vi "GetROSfromTopic.vi"(0 "Topic":string) -> (2 "ROS":T1, 3 "Nice Name":string, 4 "Node?":bool)   [LabVIEW 2016]
doc: "Gets ROS typdef from the topic name"
uses:
  _ROSControl.ctl
  _ROSDirection.ctl
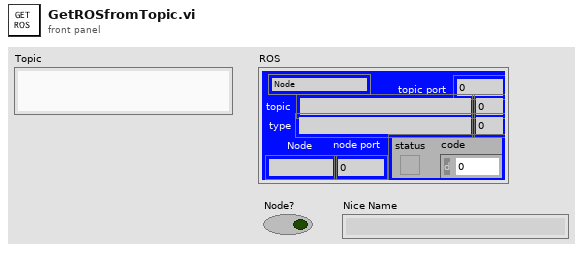
[diagram p1: front panel]
types:
  T1 = typedef "_ROSControl.ctl" = cluster{"topic port":u16, "Node":string, "topic":string, "type":string, "node port":u16, "error ":errorcluster, "Direction":T2, "Update (ms)":u16, "FIFO size":u16}
  T2 = typedef "_ROSDirection.ctl" = enum16{"Node", "Publisher", "Subscriber", "ServiceClient", "ServiceProvider"}
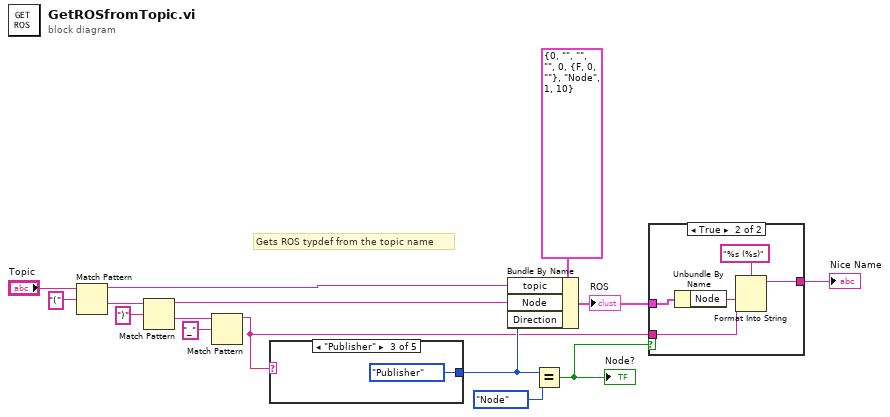
[diagram p0: block diagram]
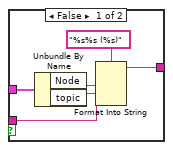
[diagram p2: hidden frame]
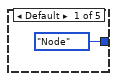
[diagram p3: hidden frame]
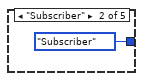
[diagram p4: hidden frame]
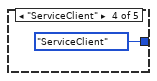
[diagram p5: hidden frame]
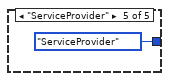
[diagram p6: hidden frame]
diagram:
  # "Gets ROS typdef from the topic name"
  n1 = Match Pattern(string="Topic", regular expression="(") -> (before substring=w5:string, after substring=w12:string)  [unwired: 1 in, 2 out]
  n2 = Match Pattern(string=w12, regular expression=")") -> (before substring=w6:string, after substring=w10:string)  [unwired: 1 in, 2 out]
  n3 = Match Pattern(string=w10, regular expression="_") -> (before substring=w4:string)  [unwired: 1 in, 3 out]
  n4 = case shown="\"Publisher\"" w4 {
    tunnel: [_ROSDirection."Node" ("Direction") _ROSDirection."Subscriber" ("Direction") _ROSDirection."Publisher" ("Direction") _ROSDirection."ServiceClient" ("Direction") _ROSDirection."ServiceProvider" ("Direction")] -> w8
    frame Default {
    }
    frame "Subscriber" {
    }
    frame "Publisher" {
    }
    frame "ServiceClient" {
    }
    frame "ServiceProvider" {
    }
  }
  n5 = Bundle By Name(cluster=T1 {"topic port"=0, "Node"="", "topic"="", "type"="", "node port"=0, "error "={"status"=FALSE, "code"=0, "source"=""}, "Direction"=enum."Node", "Update (ms)"=1, "FIFO size"=10} ("ROS"), "topic"=w5, "Node"=w6, "Direction"=w8) -> (w2:T1)
  "ROS" <- w2
  n6 = Equal?(x=w8, y=_ROSDirection."Node" ("Direction")) -> (x = y?=w1:bool)
  "Node?" <- w1
  n7 = case shown="True" w1 {
    tunnel: w4 -> [w25 w30]
    tunnel: [w24 w29] -> w3
    tunnel: w2 -> [w23 w28]
    frame False {
      n8 = Unbundle By Name(w23) -> ("Node"=w22:string, "topic"=w21:string)
      n9 = Format Into String(format string="%s%s (%s)", w22, w21, w25) -> (resulting string=w24:string)  [unwired: 2 in, 1 out]
    }
    frame True {
      n10 = Unbundle By Name(w28) -> ("Node"=w27:string)
      n11 = Format Into String(format string="%s (%s)", w27, w30) -> (resulting string=w29:string)  [unwired: 2 in, 1 out]
    }
  }
  "Nice Name" <- w3
